vi "良率計算.vi"(10 "NG":u16, 11 "OK":u16) -> (3 "良率":dbl)   [LabVIEW 2019]
panel:
  out "x/y":dbl
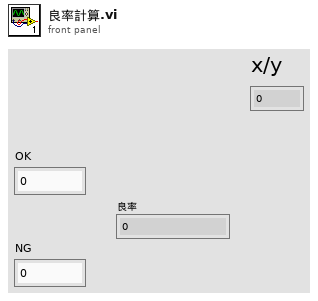
[diagram p1: front panel]
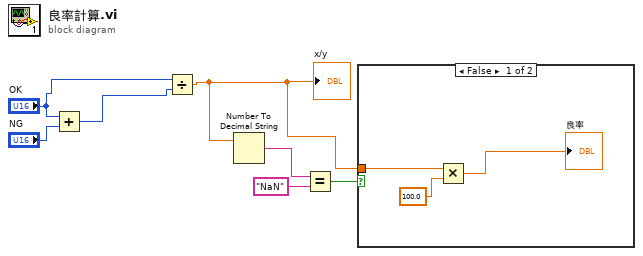
[diagram p0: block diagram]
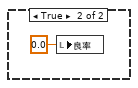
[diagram p2: hidden frame]
diagram:
  n1 = Add(x="OK", y="NG") -> (x+y=w6:u16)
  n2 = Divide(x="OK", y=w6) -> (x/y=w1:dbl)
  "x/y" <- w1
  n3 = Number To Decimal String(number=w1) -> (decimal integer string=w3:string)  [unwired: 1 in]
  n4 = Equal?(x=w3, y="NaN" ("decimal integer string")) -> (x = y?=w2:bool)
  n5 = case shown="False" w2 {
    tunnel: w1 -> [w8 _]
    frame False {
      n6 = Multiply(x=w8, y=100.0) -> (x*y=→"良率":dbl)
    }
    frame True {
      n7 = local write "良率"(0.0 ("良率")) -> ()
    }
  }
